vi "Intro.vi"() -> ()   [LabVIEW 2021]
panel:
  out "?":bool
  in  "Blank Button":bool
  in  "?":bool
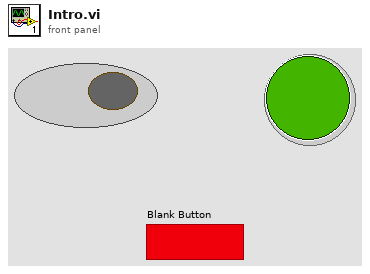
[diagram p1: front panel]
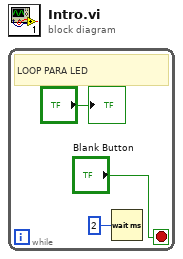
[diagram p0: block diagram]
diagram:
  n1 = while {
    stop <- "Blank Button" stop-if-true
    # "LOOP PARA LED"
    n2 = Wait (ms)(milliseconds to wait=u32 2 ("millisecond timer value")) -> ()  [unwired: 1 out]
    "?" <- "?"
  }
